vi "UserAccount_to_string.vi"(1 "Account":T1) -> (0 "String":string)   [LabVIEW 2012]
uses:
  typedef/User Accounts.ctl
panel:
  out "error out":errorcluster
  in  "error in (no error)":errorcluster
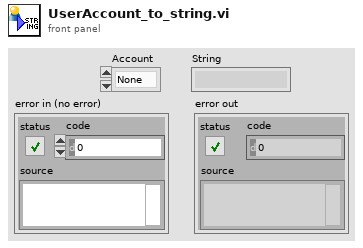
[diagram p1: front panel]
types:
  T1 = typedef "User Accounts.ctl" = enum16{"None", "User", "Admin"}
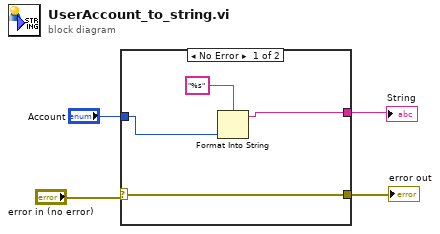
[diagram p0: block diagram]
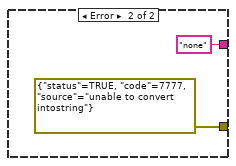
[diagram p2: hidden frame]
diagram:
  n1 = case shown="No Error" "error in (no error)" {
    selector: "error in (no error)" -> [w8 _]
    tunnel: "Account" -> [w5 _]
    tunnel: [w8 errorcluster {"status"=TRUE, "code"=7777, "source"="unable to convert intostring"} ("error IO")] -> w2
    tunnel: [w6 "none"] -> w1
    frame No Error {
      n2 = Format Into String "Format Into String"(format string="%s", w5) -> (resulting string=w6:string)  [unwired: 2 in, 1 out]
    }
    frame Error {
    }
  }
  "error out" <- w2
  "String" <- w1
